vi "ATF-Pump-DI Start.vi"(8 "error in":errorcluster, 9 "DI config":T1(array[cluster]), 11 "Refnum in":refnum<k21>) -> (0 "error out":errorcluster, 3 "Refnum out":refnum<k21>)   [LabVIEW 2022 SP3]
doc: "This VI is for start for Analog Output"
uses:
  <resource>/objmgr/daqmx.rc
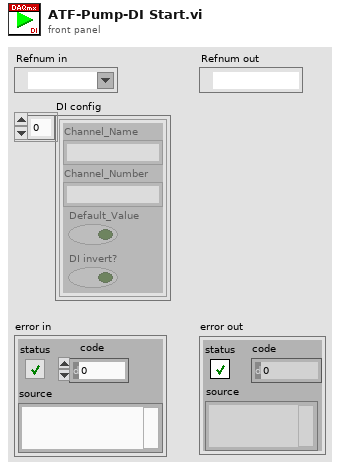
[diagram p1: front panel]
types:
  T1 = cluster{"Channel_Name":string, "Channel_Number":string, "Default_Value":bool, "DI invert?":bool}[]
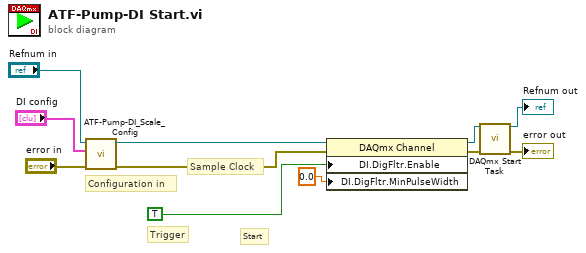
[diagram p0: block diagram]
diagram:
  # "Start"
  # "Trigger"
  # "Sample Clock"
  # "Configuration in"
  n1 = call "ATF-Pump-DI_Scale_Config.vi"("error in (no error)"="error in", "DI config"="DI config", "Refnum in"="Refnum in") -> ("error out"=w10:errorcluster, "Refnum out"=w9:refnum<k21>)  [unwired: 7 in]
  n2 = property class="DAQmx Channel"(reference=w9, error in=w10, "DI.DigFltr.Enable"=TRUE, "DI.DigFltr.MinPulseWidth"=0.0) -> (reference out=w4:refnum<k21>, error out=w3:errorcluster)
  n3 = call <vilib>:"DAQmx Start Task.vi"("task/channels in"=w4, "error in"=w3) -> ("task out"=→"Refnum out":refnum<k21>, "error out"=→"error out":errorcluster)  [unwired: 12 in]
